vi "Get Subpanel Ref.vi"(8 "error in (no error)":errorcluster, 11 "Owner VI in":refnum<vi>) -> (0 "error out":errorcluster, 2 "SubPanel out":refnum<vi>)   [LabVIEW 2019, in "gRPC Scripting Tools.lvlib"]
uses:
  gRPC Scripting Tools.lvlib
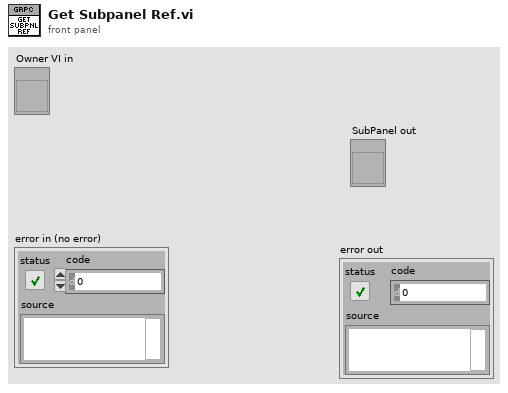
[diagram p1: front panel]
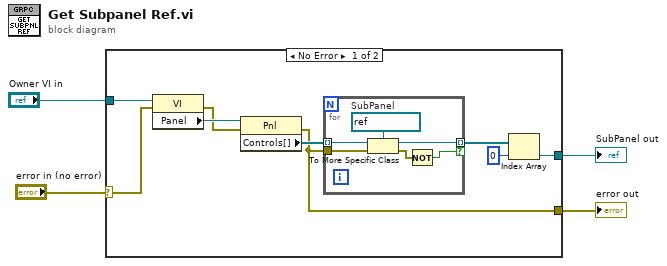
[diagram p0: block diagram]
diagram:
  n1 = case shown="No Error" "error in (no error)" {
    selector: "error in (no error)" -> [w7 w20]
    tunnel: [w13 _] -> w4
    tunnel: "Owner VI in" -> [w8 _]
    tunnel: [w5 w20] -> w1
    frame No Error {
      n2 = property class="VI"(reference=w8, error in=w7) -> (error out=w6:errorcluster, "Panel"=w9:refnum<vi>)  [unwired: 1 out]
      n3 = property class="Pnl"(reference=w9, error in=w6) -> (error out=w5:errorcluster, "Controls[]"=w10:refnum<vi>[])  [unwired: 1 out]
      n4 = for {
        tunnel: w10 -> [w18] mode=indexing
        tunnel: [w17] -> w11 mode=indexing if=w15
        tunnel: w5 -> [w14]
        w19 = refnum<vi> refnum  # SubPanel
        n5 = To More Specific Class(target class=w19, reference=w18, error in=w14) -> (specific class reference=w17:refnum<vi>, error out=w16:errorcluster)
        n6 = Not(x=w16) -> (.not. x?=w15:bool)
      }
      n7 = Index Array(array=w11, index=0) -> (element=w13:refnum<vi>)
    }
    frame Error {
    }
  }
  "SubPanel out" <- w4
  "error out" <- w1
